vi "testprops mod cfg.vi"() -> ()   [LabVIEW 2013, in "TBM Tests.lvlib"]
uses:
  TBM Tests.lvlib
  module configuration/TBM module configuration.lvclass
  module configuration/timing source.ctl
panel:
  out "no err":errorcluster
  out "count ok":bool
  out "target support ok":bool
  out "no default dynamism":bool
  out "type support ok":bool
  out "runtime class ok":bool
  out "err 538305":errorcluster
  out "err 538305":errorcluster
  out "source=none":bool
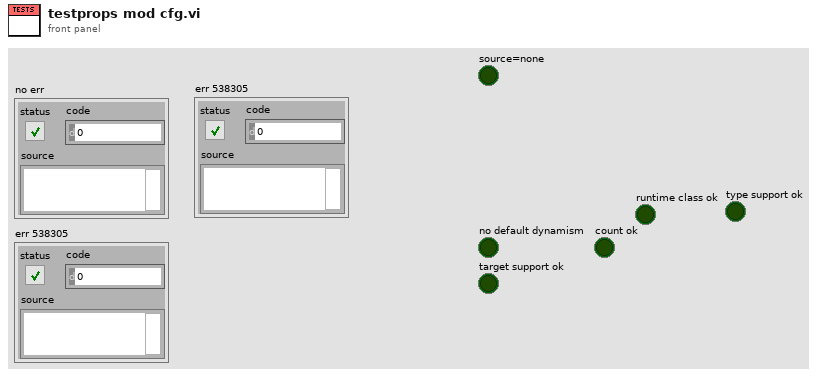
[diagram p1: front panel]
types:
  T1 = typedef "TBM module configuration.lvclass/timing source.ctl" = enum16{"None", "Custom Timing Source", "1 kHz Clock", "1 MHz Clock", "Synchronize to Scan Engine"}
  T2 = typedef "TBM configuration.lvclass/Target Types.ctl" = enum16{"Windows", "Mac", "Linux", "Linux RT ARM", "VxWorks", "Pharlap", "Other", "Linux RT x64"}
  T3 = typedef "tag bus.lvlib/tag descriptor.lvclass/Data Type.ctl" = enum16{"Double", "Single", "I64", "I32", "I16", "I8", "U64", "U32", "U16", "U8", "Boolean", "String", "Array of Double", "Array of Single", "Array of I64", "Array of I32", "Array of I16", "Array of I8", "Array of U64", "Array of U32", "Array of U16", "Array of U8", "Array of Boolean", "Array of String"}
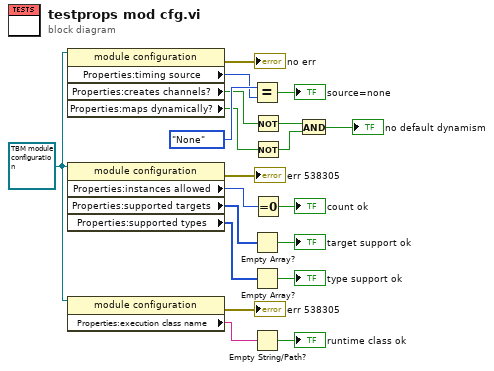
[diagram p0: block diagram]
diagram:
  w5 = refnum<class "TBM module configuration.lvclass"> refnum ("module configuration")
  n1 = property class="module configuration"(reference=w5) -> (error out=→"no err":errorcluster, "Properties:timing source"=w4:T1, "Properties:creates channels?"=w1:bool, "Properties:maps dynamically?"=w2:bool)  [unwired: 1 in, 1 out]
  n2 = property class="module configuration"(reference=w5) -> (error out=→"err 538305":errorcluster, "Properties:instances allowed"=w7:i32, "Properties:supported targets"=w9:T2[], "Properties:supported types"=w14:T3[])  [unwired: 1 in, 1 out]
  n3 = property class="module configuration"(reference=w5) -> (error out=→"err 538305":errorcluster, "Properties:execution class name"=w16:string)  [unwired: 1 in, 1 out]
  n4 = Equal?(x=timing_source."None", y=w4) -> (x = y?=→"source=none":bool)
  n5 = Empty Array?(array=w9) -> (empty?=→"target support ok":bool)
  n6 = Empty Array?(array=w14) -> (empty?=→"type support ok":bool)
  n7 = Empty String/Path?(string/path=w16) -> (empty?=→"runtime class ok":bool)
  n8 = Not(x=w1) -> (.not. x?=w10:bool)
  n9 = Not(x=w2) -> (.not. x?=w12:bool)
  n10 = Equal To 0?(x=w7) -> (x = 0?=→"count ok":bool)
  n11 = And(x=w10, y=w12) -> (x .and. y?=→"no default dynamism":bool)
